vi "SPI1_DEMO_TLA2518.vi"() -> ()   [LabVIEW 2017]
uses:
  Saldigi_protocol_library.lvlibp/HAL/HAL_version_typedef.ctl
  Saldigi_protocol_library.lvlibp/SPI1_bitstream/SPI1_typedef.ctl
  Saldigi_protocol_library.lvlibp/Drivers/TLA2518_typedef.ctl
  Saldigi_protocol_library.lvlibp
panel:
  in  "Version":T1=enum."FTn232H"
  in  "Parameter string":string(combo)="FTERYEPB"
  in  "MISO IO1 channel name":string(combo)="D3"
  in  "CLK channel name":string(combo)="D0"
  in  "MOSI IO0 channel name":string(combo)="D1"
  in  "-CS channel name":string(combo)="D6"
  in  "output rate":dbl=20000000.0 format="%^#_6g"
  out "iteration#":i32
  in  "stop":bool
  out "TLA2518 Register value out":u8 format="%.0x"
  out "error out":errorcluster
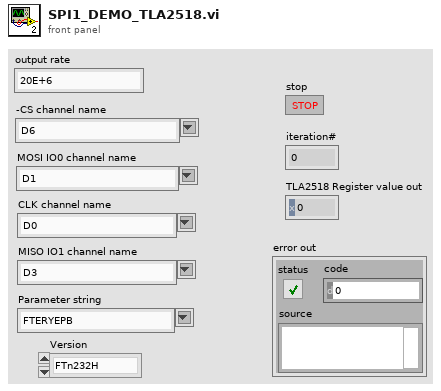
[diagram p1: front panel]
types:
  T1 = typedef "Saldigi_protocol_library.lvlibp/HAL_version_typedef.ctl" = enum16{"DAQmx V1", "DAQmx V2", "FTn232H", "BSCAN V1", "DAQmx V1.1", "DAQmx V2.1", "J-LINK BSCAN", "BSCAN V2"}
  T2 = typedef "Saldigi_protocol_library.lvlibp/SPI1_typedef.ctl" = cluster{"MOSI padded":bool[], "CLK padded":bool[], "-CS padded":bool[], "String array":string[], "clocked bits":i32, "output rate":dbl, "MOSI IO0 channel name":string, "CLK channel name":string, "MISO IO1 channel name":string, "Parameter string":string, "-CS channel name":string, "SPI mode":enum16{"MODE 0", "MODE 1", "MODE 2", "MODE 3"}, "Version":T1}
  T3 = typedef "Saldigi_protocol_library.lvlibp/TLA2518_typedef.ctl" = enum16{"SYSTEM_STATUS", "GENERAL_CFG", "DATA_CFG", "OSR_CFG", "OPMODE_CFG", "PIN_CFG", "NA6", "GPIO_CFG", "NA8", "GPO_DRIVE_CFG", "NA_A", "GPO_VALUE", "NA_C", "GPI_VALUE", "NA_E", "NA_F", "SEQUENCE_CFG", "CHANNEL_SEL", "AUTO_SEQ_CH_SEL"}
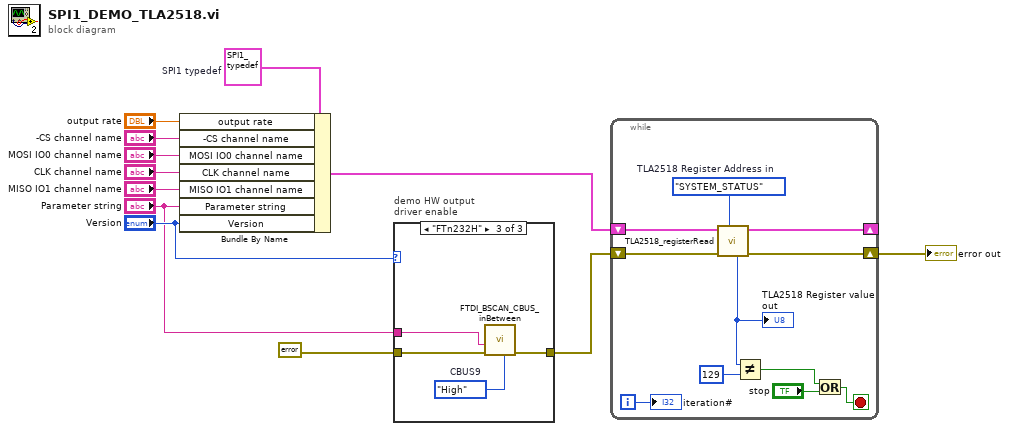
[diagram p0: block diagram]
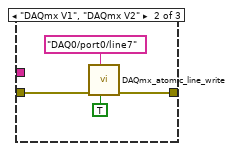
[diagram p3: hidden frame]
diagram:
  w4 = T2 {"MOSI padded"=[], "CLK padded"=[], "-CS padded"=[], "String array"=[], "clocked bits"=0, "output rate"=1000000.0, "MOSI IO0 channel name"="DAQ0/port0/line1", "CLK channel name"="DAQ0/port0/line0", "MISO IO1 channel name"="DAQ0/port0/line3", "Parameter string"="PFI5", "-CS channel name"="DAQ0/port0/line6", "SPI mode"=enum."MODE 0", "Version"=enum."DAQmx V1"}  # SPI1 typedef
  n1 = Bundle By Name(cluster=w4, "output rate"="output rate", "-CS channel name"="-CS channel name", "MOSI IO0 channel name"="MOSI IO0 channel name", "CLK channel name"="CLK channel name", "MISO IO1 channel name"="MISO IO1 channel name", "Parameter string"="Parameter string", "Version"="Version") -> (w3:T2)
  n2 = case "demo HW output\ndriver enable" shown="\"FTn232H\"" "Version" {
    tunnel: errorcluster {"status"=FALSE, "code"=0, "source"=""} ("error in") -> [w13 w15 w21]
    tunnel: [w13 w14 w20] -> w11
    tunnel: "Parameter string" -> [_ _ w18]
    frame Default {
    }
    frame "DAQmx V1", "DAQmx V2" {
      n3 = call "DAQmx_atomic_line_write.vi"("line state in"=TRUE, "dev/port/line in"="DAQ0/port0/line7" ("demo HW output\ndriver enable"), "error in"=w15) -> ("error out"=w14:errorcluster)  [unwired: 8 in]
    }
    frame "FTn232H" {
      w19 = enum16{"Low", "High", "Input"}."High"  # CBUS9
      n4 = call "FTDI_BSCAN_CBUS_inBetween.vi"("CBUS9"=w19, "error in"=w21, "parameter string in (SerNo)"=w18) -> ("error out"=w20:errorcluster)  [unwired: 8 in]
    }
  }
  n5 = while {
    shift-right: [w30] -> w10
    shift-left: w11 -> [w31]
    shift-right: [w23] -> _
    shift-left: w3 -> [w32]
    i -> [w22]
    stop <- w26 stop-if-true
    w29 = TLA2518_typedef."SYSTEM_STATUS"  # TLA2518 Register Address in
    n6 = call "TLA2518_registerRead.vi"("TLA2518 Register Address in"=w29, "error in"=w31, "SPI1 typedef in"=w32) -> ("error out"=w30:errorcluster, "SPI1 typedef out"=w23:T2, "TLA2518 Register value out"=w28:u8)  [unwired: 6 in]
    "TLA2518 Register value out" <- w28
    n7 = Not Equal?(x=w28, y=u8 129) -> (x != y?=w25:bool)
    n8 = Or(x=w25, y="stop") -> (x .or. y?=w26:bool)
    "iteration#" <- w22
  }
  "error out" <- w10
